vi "Read ODrive return data.vi"(8 "error in (no error)":errorcluster, 11 "Refnum in":refnum<k20>) -> (0 "error out":errorcluster, 3 "Refnum out":refnum<k20>)   [LabVIEW 2016]
uses:
  Shared resoruces/gear.vi
  <vilib>/Utility/error.llb/Error Cluster From Error Code.vi
  <vilib>/rvi/errors/niLvFpgaAdjustHostInterfaceError.vi
  Shared resoruces/ODrive State and Info.vi
  Shared resoruces/Navigation Variables.vi
  <vilib>/rvi/interface/nirviReadWriteControl/nirviReadWriteControl.xnode
  NiFpgaLv.dll
  <vilib>/rvi/interface/Simulation/niFpgaSimulationCallBeginRW.vi
  Shared resoruces/Shared resources RT.lvlib
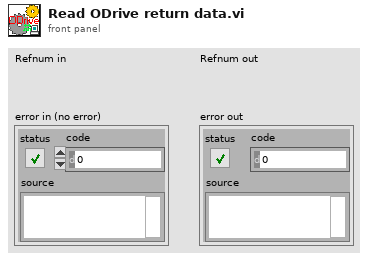
[diagram p1: front panel]
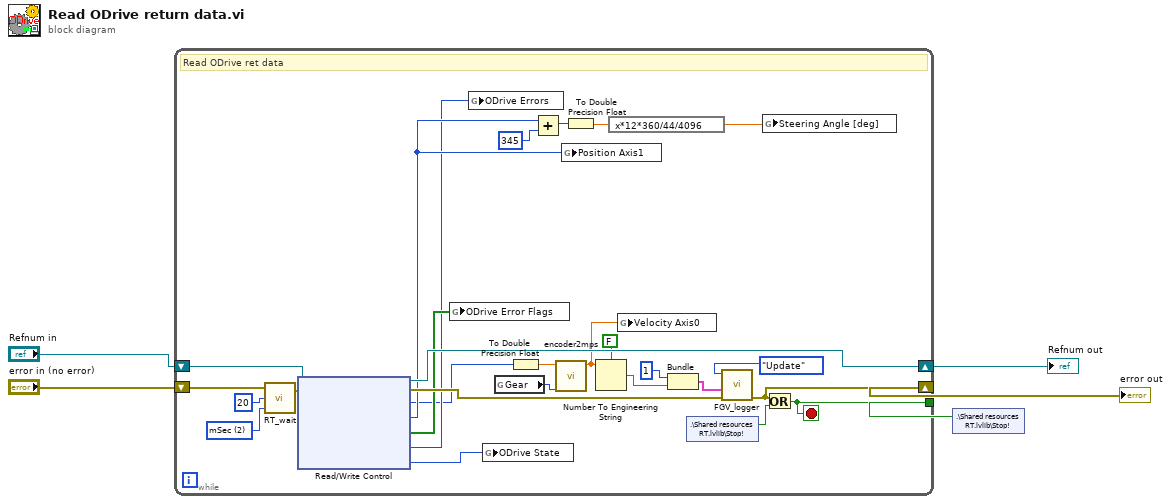
[diagram p0: block diagram]
diagram:
  n1 = while {
    shift-right: [w32] -> w5
    shift-left: "Refnum in" -> [w31]
    shift-right: [w12] -> w1
    shift-left: "error in (no error)" -> [w30]
    tunnel: [w25] -> w2
    stop <- w25 stop-if-true
    w27 = u16 2 items=["Ticks", "uSec", "mSec"] ("Counter Units")
    # "Read ODrive ret data"
    n2 = call "RT_wait.vi"("Counter Units"=w27, "Count(mSec)"=u32 20, "error in (no error)"=w30) -> ("error out"=w29:errorcluster)  [unwired: 1 in, 1 out]
    n3 = xnode "Read/Write Control"("FPGA VI Reference In"=w31, "error in"=w29) -> ("FPGA VI Reference Out"=w32:refnum<k20>, "error out"=w21:errorcluster, "Velocity Axis0"=w9:i16, "Position Axis1"=w16:i16, "ODrive Error Flags"=w17:bool[], "ODrive Errors"=w15:u32, "ODrive State"=w14:u8)
    n4 = global write "ODrive State and Info.vi" "ODrive Error Flags"(w17) -> ()
    n5 = global write "ODrive State and Info.vi" "ODrive Errors"(w15) -> ()
    n6 = global write "ODrive State and Info.vi" "ODrive State"(w14) -> ()
    n7 = global read "gear.vi" "Gear"() -> (w11:enum16{"7", "6", "5", "4", "3", "2", "1"})
    n8 = To Double Precision Float(number=w9) -> (double precision float=w10:dbl)
    n9 = Add(x=w16, y=i16 345 ("hi")) -> (x+y=w19:i16)
    n10 = call "encoder2mps.vi"("Gear"=w11, "encoderSpeed"=w10) -> ("realVelocity"=w6:dbl)  [unwired: 9 in]
    n11 = global write "ODrive State and Info.vi" "Position Axis1"(w16) -> ()
    n12 = To Double Precision Float(number=w19) -> (double precision float=w18:dbl)
    n13 = Number To Engineering String(1:FALSE ("use system decimal point (T)"), 4:w6) -> (0:w7:string)  [unwired: 2 in]
    n14 = expression code="x*12*360/44/4096"(w18) -> (w13:dbl)
    n15 = global write "ODrive State and Info.vi" "Velocity Axis0"(w6) -> ()
    n16 = Bundle(1, w7) -> (w23:cluster{i32, string})  [unwired: 1 in]
    n17 = shared-variable ".\\Shared resources RT.lvlib\\Stop!"() -> (w26:bool)  [unwired: 1 in, 1 out]
    n18 = call "FGV_logger.vi"("error in"=w21, 9:w23, "Command"=enum16{"Update", "Log", "Init"}."Update") -> ("error out"=w12:errorcluster)  [unwired: 8 in]
    n19 = global write "Navigation Variables.vi" "Steering Angle [deg]"(w13) -> ()
    n20 = Or(x=w12, y=w26) -> (x .or. y?=w25:bool)
  }
  "Refnum out" <- w5
  "error out" <- w1
  n21 = shared-variable ".\\Shared resources RT.lvlib\\Stop!"(w2) -> ()  [unwired: 1 in, 1 out]
